vi "RFSA_Analysis_Control.vi"(8 "error in (no error)":errorcluster, 11 "Message_Queues":T1) -> (0 "error out":errorcluster)   [LabVIEW 2014]
uses:
  02_Controls/Message_Queues.ctl
  02_Controls/Message_Data_Ctl.ctl
  15_DataManagement/Analysis_Parameters.ctl
  <vilib>/measure/masml.llb/ma_sml_Averaging Parameters.ctl
  <vilib>/measure/masml.llb/ma_sml_Averaging Settings.ctl
  <vilib>/addons/Spectral Measurements Toolset/LVSupport/SMT BZ spectrum settings.ctl
  <vilib>/addons/Spectral Measurements Toolset/LVSupport/SMT Zoom Power Spectrum (Complex Input).vi
  <vilib>/addons/Spectral Measurements Toolset/niSMT.lvlib
  <vilib>/measure/NI_MAPro.lvlib
panel:
  out "Waveform Graph 2":cluster{"f0":dbl, "df":dbl, "data":dbl[]}(graph)
  out "size(s)":i32
  out "power in adjacent channels":dbl[](array[numeric])
  out "power in central channel":dbl
  out "Waveform Graph":cluster{"t0":dbl, "dt":dbl, "Y":dbl[]}[](graph)
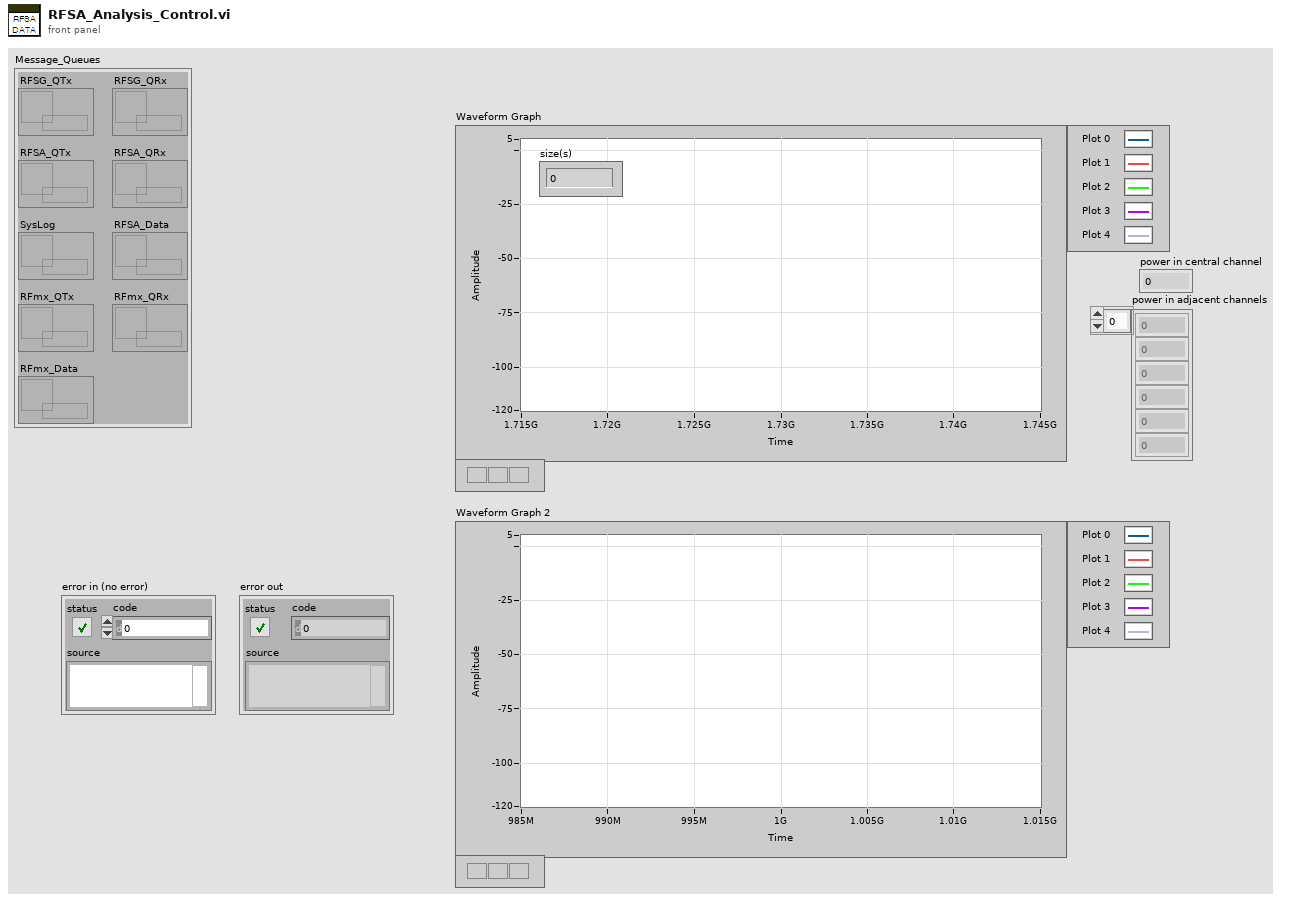
[diagram p1: front panel]
types:
  T1 = typedef "Message_Queues.ctl" = cluster{"RFSG_QTx":refnum<queue>, "RFSG_QRx":refnum<queue>, "RFSA_QTx":refnum<queue>, "RFSA_QRx":refnum<queue>, "SysLog":refnum<queue>, "RFSA_Data":refnum<queue>, "RFmx_QTx":refnum<queue>, "RFmx_QRx":refnum<queue>, "RFmx_Data":refnum<queue>}
  T2 = typedef "Analysis_Parameters.ctl" = cluster{"carrier frequency":dbl, "IQ rate (S/s)":dbl, "samples per record":i64, "Signal Bandwidth (Hz)":dbl, "Resolution Bandwidth (Hz)":dbl, "Ref ch Bandwidth (Hz)":dbl, "Offset_Freq(Hz)":dbl[], "Integration_Bandwidth(Hz)":dbl[]}
  T3 = enum16{"V", "V^2", "W", "dBm", "dBW", "dBV", "dBmV", "dBuV"}
  T4 = cluster{"type":enum16{"real", "complex modulated"}, "frequency shift":dbl}
  T5 = typedef "niSMT.lvlib/SMT BZ spectrum settings.ctl" = cluster{"center frequency":dbl, "span":dbl, "resolution bandwidth":dbl}
  T6 = typedef "NI_MAPro.lvlib/ma_sml_Averaging Parameters.ctl" = cluster{"averaging type":enum16{"no averaging", "vector averaging", "RMS averaging", "peak hold"}, "averaging settings":T7}
  T7 = typedef "NI_MAPro.lvlib/ma_sml_Averaging Settings.ctl" = cluster{"weighting type":enum16{"linear", "exponential"}, "weighting settings":cluster{"size":dbl, "linear weighting mode":enum16{"one shot", "auto restart one shot", "moving average", "continuous"}}}
  T8 = cluster{"units":enum16{"V", "V^2", "W", "dBm", "dBW", "dBV", "dBmV", "dBuV"}, "peak scaling":enum16{"rms", "pk"}, "psd?":bool, "impedance(ohm)":dbl}
  T9 = cluster{"window":enum16{"None ", "Hanning", "Hamming", "Blackman-Harris", "Exact Blackman", "Blackman", "Flat Top", "4 Term B-Harris ", "7 Term B-Harris", "Low Sidelobe"}, "spectral lines":i32, "effective band specification":cluster{"fl":dbl, "fh":dbl}, "RBW definition":enum16{"3dB", "6dB", "ENBW", "bin width"}}
  T10 = typedef "niSMT.lvlib/SMT zoom settings.ctl" = cluster{"zoom FFT settings":T11, "frequency shift":dbl, "data format":enum16{"real", "complex modulated (array)", "complex modulated (interleaved)"}}
  T11 = typedef "NI_MAPro.lvlib/ma_sml_ND Zoom FFT Settings.ctl" = cluster{"zoom settings":cluster{"center frequency":dbl, "zoom":i32, "trim":dbl}, "FFT settings":cluster{"window":u16, "FFT size":i32}}
  T12 = typedef "NI_MAPro.lvlib/ma_sml_Spectral Info.ctl" = cluster{"spectrum type":enum16{"FFT Spectrum [complex]", "Amplitude [Magnitude]", "Power [Magnitude^2]", "Cross Spectrum [complex]", "Frequency Response [Complex]"}, "linear/dB":enum16{"linear", "dB"}, "window":u16, "window size":i32, "FFT size":i32}
  T13 = typedef "NI_MAPro.lvlib/ma_sml_Spectrum Cluster (real).ctl" = cluster{"f0":dbl, "df":dbl, "spectrum":dbl[]}
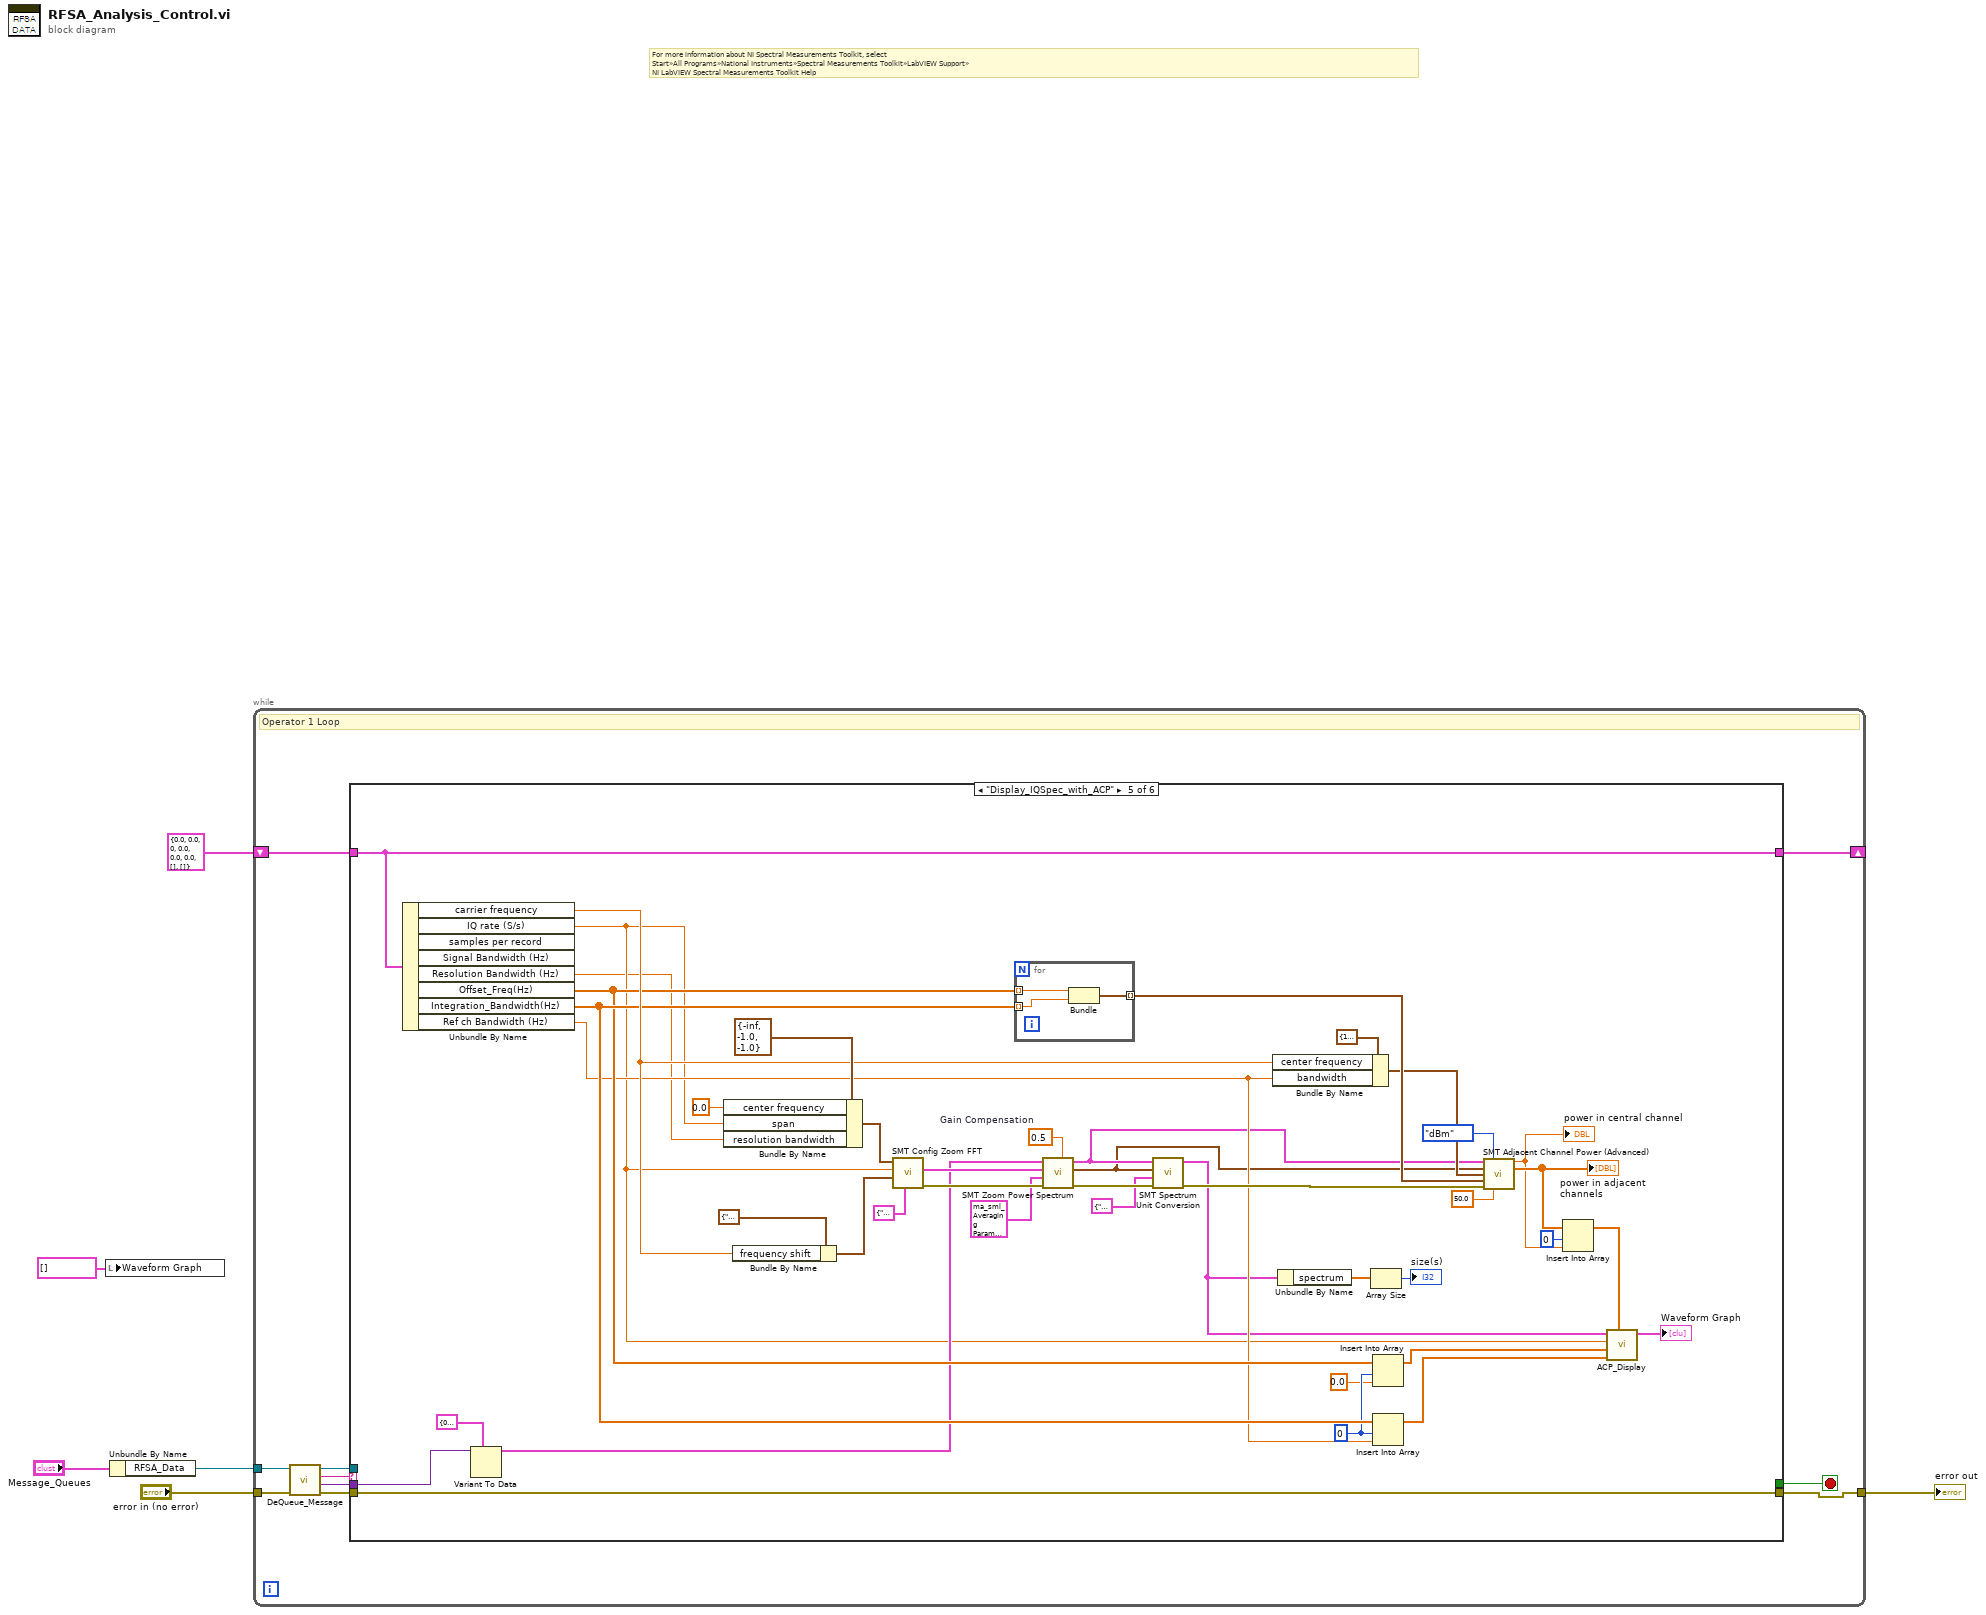
[diagram p0: block diagram]
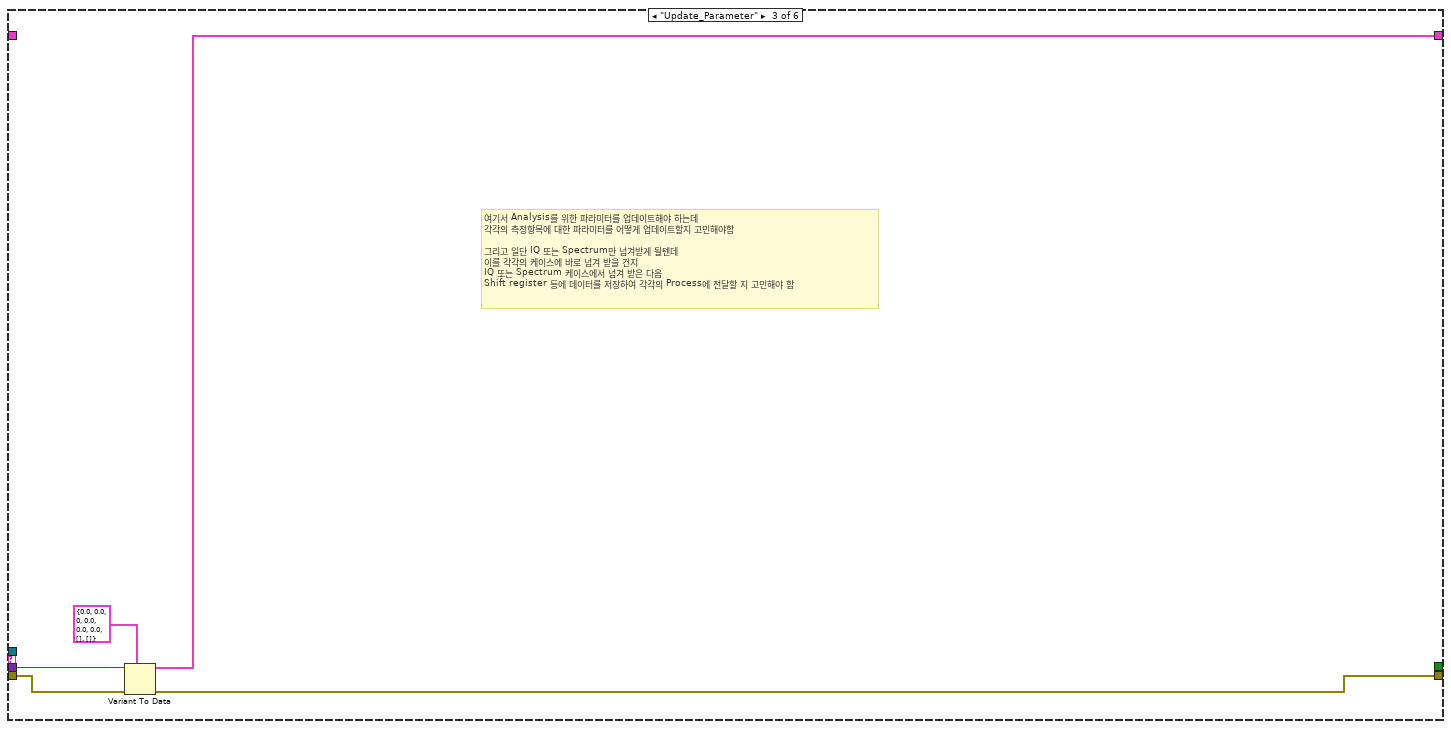
[diagram p4: hidden frame]
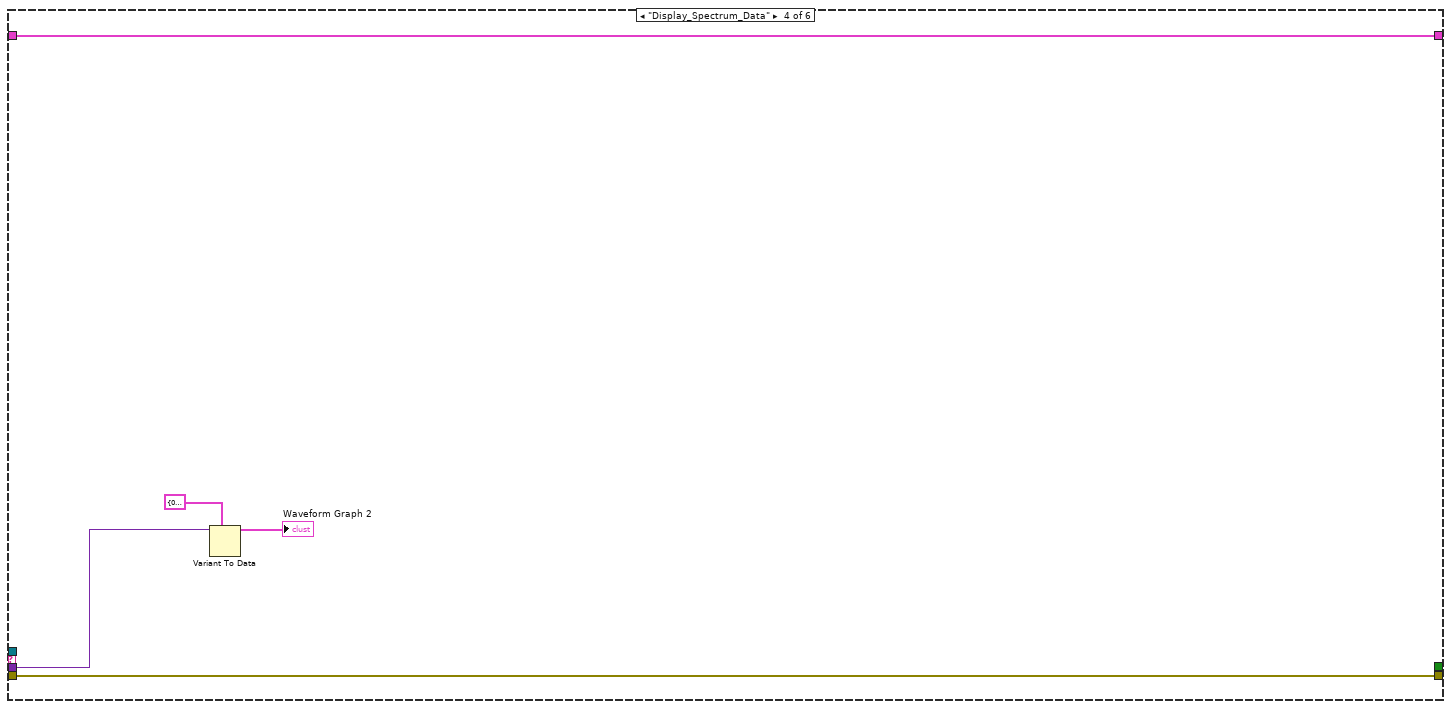
[diagram p5: hidden frame]
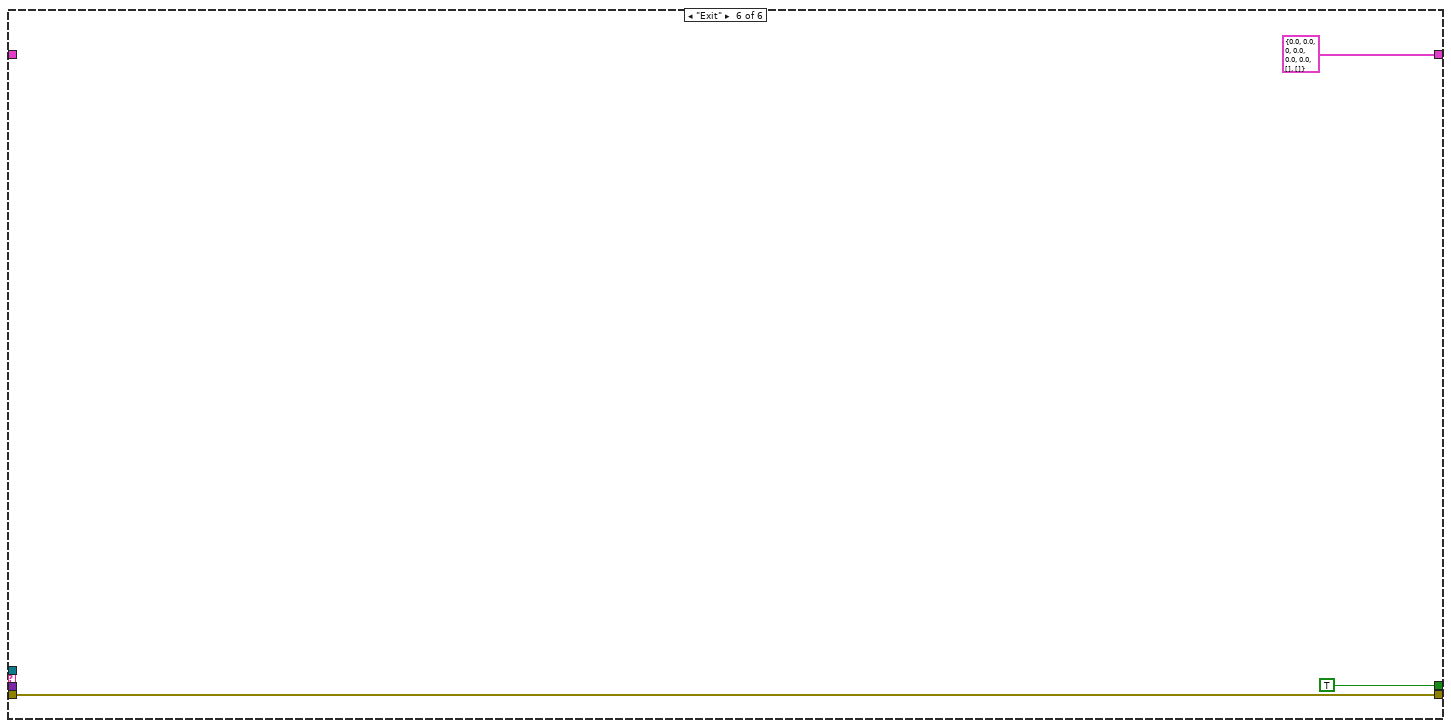
[diagram p6: hidden frame]
diagram:
  # "For more information about NI Spectral Measurements Toolkit, select \nStart»All Programs»National Instruments»Spectral Measurements Toolkit»LabVIEW Support»\nNI LabVIEW Spectral Measurements Toolkit Help"
  n1 = local write "Waveform Graph"(cluster{"t0":dbl, "dt":dbl, "Y":dbl[]}[] [] ("Waveform Graph")) -> ()
  n2 = Unbundle By Name("Message_Queues") -> ("RFSA_Data"=w4:refnum<queue>)
  n3 = while {
    tunnel: "error in (no error)" -> [w16]
    tunnel: [w10] -> w5
    tunnel: w4 -> [w9]
    shift-right: [w8] -> _
    shift-left: T2 {"carrier frequency"=0.0, "IQ rate (S/s)"=0.0, "samples per record"=0, "Signal Bandwidth (Hz)"=0.0, "Resolution Bandwidth (Hz)"=0.0, "Ref ch Bandwidth (Hz)"=0.0, "Offset_Freq(Hz)"=[], "Integration_Bandwidth(Hz)"=[]} ("Analysis_Parameters") -> [w7]
    stop <- w11 stop-if-true
    # "Operator 1 Loop"
    n4 = call "DeQueue_Message.vi"("error in (no error)"=w16, "Message_Queue"=w9) -> ("error out"=w12:errorcluster, "Message Data"=w14:variant, "Message"=w15:string, "Dup_Message_Queue"=w13:refnum<queue>)  [unwired: 6 in]
    n5 = case shown="\"Display_IQSpec_with_ACP\"" w15 {
      tunnel: w14 -> [_ _ w25 w29 w72 _]
      tunnel: w13 -> [_ _ _ _ _ _]
      tunnel: w12 -> [w18 w20 w22 w30 w73 w78]
      tunnel: [_ _ _ _ _ TRUE] -> w11
      tunnel: [w18 w20 w21 w30 w73 w78] -> w10
      tunnel: [w17 w19 w23 w28 w63 T2 {"carrier frequency"=0.0, "IQ rate (S/s)"=0.0, "samples per record"=0, "Signal Bandwidth (Hz)"=0.0, "Resolution Bandwidth (Hz)"=0.0, "Ref ch Bandwidth (Hz)"=0.0, "Offset_Freq(Hz)"=[], "Integration_Bandwidth(Hz)"=[]} ("Analysis_Parameters")] -> w8
      tunnel: w7 -> [w17 w19 _ w28 w63 _]
      frame "Nothing", Default {
      }
      frame "===== DisplayData =====" {
      }
      frame "Update_Parameter" {
        # "여기서 Analysis를 위한 파라미터를 업데이트해야 하는데\n각각의 측정항목에 대한 파라미터를 어떻게 업데이트할지 고민해야함\n\n그리고 일단 IQ 또는 Spectrum만 넘겨받게 될텐데\n이를 각각의 케이스에 바로 넘겨 받을 건지\nIQ 또는 Spectrum 케이스에서 넘겨 받은 다음\nShift register 등에 데이터를 저장하여 각각의 Process에 전달할 지 고민해야 함"
        n6 = Variant To Data(error in=w22, type=T2 {"carrier frequency"=0.0, "IQ rate (S/s)"=0.0, "samples per record"=0, "Signal Bandwidth (Hz)"=0.0, "Resolution Bandwidth (Hz)"=0.0, "Ref ch Bandwidth (Hz)"=0.0, "Offset_Freq(Hz)"=[], "Integration_Bandwidth(Hz)"=[]} ("Analysis_Parameters"), Variant=w25) -> (data=w23:T2, error out=w21:errorcluster)
      }
      frame "Display_Spectrum_Data" {
        n7 = Variant To Data(type=cluster{"f0":dbl, "df":dbl, "data":dbl[]} {"f0"=0.0, "df"=0.0, "data"=[]} ("power spectrum"), Variant=w29) -> (data=→"Waveform Graph 2":cluster{"f0":dbl, "df":dbl, "data":dbl[]})  [unwired: 1 in, 1 out]
      }
      frame "Display_IQSpec_with_ACP" {
        w47 = 0 ("index")
        w70 = 0.5  # Gain Compensation
        n8 = Unbundle By Name(w63) -> ("carrier frequency"=w51:dbl, "IQ rate (S/s)"=w32:dbl, "Resolution Bandwidth (Hz)"=w31:dbl, "Offset_Freq(Hz)"=w48:dbl[], "Integration_Bandwidth(Hz)"=w49:dbl[], "Ref ch Bandwidth (Hz)"=w39:dbl)  [unwired: 2 out]
        n9 = Variant To Data(type=cluster{"t0":dbl, "dt":dbl, "Y":cdb[]} {"t0"=0.0, "dt"=0.0, "Y"=[]} ("data"), Variant=w72) -> (data=w33:cluster{"t0":dbl, "dt":dbl, "Y":cdb[]})  [unwired: 1 in, 1 out]
        n10 = Bundle By Name(cluster=T5 {"center frequency"=-inf, "span"=-1.0, "resolution bandwidth"=-1.0} ("spectrum settings"), "center frequency"=0.0, "span"=w32, "resolution bandwidth"=w31) -> (w61:T5)
        n11 = Bundle By Name(cluster=T4 {"type"=enum."complex modulated", "frequency shift"=0.0} ("input signal settings"), "frequency shift"=w51) -> (w59:T4)
        n12 = call <vilib>:"SMT Config Zoom FFT.vi"("advanced settings"=T9 {"window"=enum."7 Term B-Harris", "spectral lines"=-1, "effective band specification"={"fl"=0.0, "fh"=0.5}, "RBW definition"=enum."3dB"}, "input signal settings"=w59, "fs"=w32, "spectrum settings"=w61) -> ("error out"=w66:errorcluster, "SMT zoom settings"=w65:T10)  [unwired: 1 in, 5 out]
        n13 = for {
          tunnel: w48 -> [w76] mode=indexing
          tunnel: w49 -> [w75] mode=indexing
          tunnel: [w74] -> w57 mode=indexing
          n14 = Bundle("Numeric"=w76, "Numeric"=w75) -> (w74:cluster{"Numeric":dbl, "Numeric":dbl})  [unwired: 1 in]
        }
        n15 = call-poly <vilib>:"SMT Zoom Power Spectrum.vi"("gain compensation"=w70, "error in (no error)"=w66, "averaging parameters"=T6 {"averaging type"=enum."no averaging", "averaging settings"={"weighting type"=enum."linear", "weighting settings"={"size"=10.0, "linear weighting mode"=enum."moving average"}}}, "SMT zoom settings"=w65, "signal in"=w33) -> ("error out"=w69:errorcluster, "spectral info"=w34:T12, "power spectrum"=w35:T13)  [unwired: 1 in, 3 out]
        n16 = call <vilib>:"SMT Spectrum Unit Conversion.vi"("error in (no error)"=w69, "unit conversion settings"=T8 {"units"=enum."dBm", "peak scaling"=enum."rms", "psd?"=FALSE, "impedance(ohm)"=50.0} ("Unit conversion settings"), "spectral info in"=w34, "power spectrum"=w35) -> ("error out"=w56:errorcluster, "unit converted spectrum"=w36:cluster{"f0":dbl, "df":dbl, "spectrum":dbl[]})  [unwired: 6 out]
        n17 = Bundle By Name(cluster=cluster{"center frequency":dbl, "bandwidth":dbl} {"center frequency"=1000000000.0, "bandwidth"=9000000.0} ("center channel specification"), "center frequency"=w51, "bandwidth"=w39) -> (w52:cluster{"center frequency":dbl, "bandwidth":dbl})
        n18 = Unbundle By Name(w36) -> ("spectrum"=w38:dbl[])
        n19 = Array Size(array=w38) -> (size(s)=→"size(s)":i32)
        n20 = Insert Into Array(array=w48, index=w47, new element=0.0 ("new element/subarray")) -> (w45:dbl[])
        n21 = Insert Into Array(array=w49, index=w47, new element=w39) -> (w44:dbl[])
        n22 = call <vilib>:"SMT Adjacent Channel Power (Advanced).vi"("power spectrum"=w35, "units"=T3."dBm", "spectral info"=w34, "center channel specification"=w52, "adjacent channel specifications"=w57, "error in (no error)"=w56, "impedance (ohm)"=50.0) -> ("power in central channel"=w42:dbl, "power in adjacent channels"=w43:dbl[])  [unwired: 5 in, 2 out]
        "power in central channel" <- w42
        "power in adjacent channels" <- w43
        n23 = Insert Into Array(array=w43, index=0, new element=w42) -> (w40:dbl[])
        n24 = call "ACP_Display.vi"("ACP_Values"=w40, "Int_Bandwidth"=w44, "Offsets"=w45, "SignalBandwidth"=w32, "Input_Waveform"=w36) -> ("Waveform Graph 2"=→"Waveform Graph":cluster{"t0":dbl, "dt":dbl, "Y":dbl[]}[])  [unwired: 6 in]
      }
      frame "Exit" {
      }
    }
  }
  "error out" <- w5
